vi "dI-dV(V)_MFLI_MF-MD_K3636B_measureX_PK_V4.0_withaveraging_copy.vi"() -> ()   [LabVIEW 2016]
uses:
  Labview Drivers/MFLI/LabOneLabVIEW-22.02.26577/LabOneLabVIEW-22.02.26577/Zurich Instruments LabOne/Public/Data/ziTypeDemodSampleSingle.ctl
  Application/Labview Drivers/Keithley 2600 Series/Public/Configure/Source/Configure Source (Limit).vi
  Application/Labview Drivers/Keithley 2600 Series/Public/Configure/Source/Configure Source (Range).vi
  Labview Drivers/MFLI/LabOneLabVIEW-22.02.26577/LabOneLabVIEW-22.02.26577/Zurich Instruments LabOne/Public/Configure/ziSetValueDouble.vi
  Labview Drivers/MFLI/LabOneLabVIEW-22.02.26577/LabOneLabVIEW-22.02.26577/Zurich Instruments LabOne/Public/Configure/ziGetValueDemodSampleEx.vi
  Labview Drivers/MFLI/LabOneLabVIEW-22.02.26577/LabOneLabVIEW-22.02.26577/Zurich Instruments LabOne/Zurich Instruments LabOne.lvlib
  Application/Labview Drivers/Keithley 2600 Series/Keithley 2600 Series.lvlib
panel:
  in  "MFLI Average":i32=50
  in  "MFLI Autorange":bool
  in  "Resistance used for DC (ohm)":dbl=2000000.0 format="%#_13g"
  in  "DC Current Limit (A)":dbl=0.001 format="%#_13g"
  in  "Keithley 2636B (channelA)":refnum<visa-resource-name>="GPIB0::26::INSTR"
  in  "DC Voltage averaging":dbl=10.0 format="%#_13g"
  out "Demod Sample Out 2":T1={"Timestamps (ticks)"=44415505503230, "X (Vrms)"=5.270432882217543e-11, "Y (Vrms)"=-1.265296628024292e-11, "Osc Phase (deg)"=0.033939324931969814, "Freq (Hz)"=7.919000069023241, "DIO"=0, "AuxIn0 (V)"=-0.16198342631105334, "AuxIn1 (V)"=0.0003336581285111606, "Trigger"=768}
  out "Demod Sample Out":T1={"Timestamps (ticks)"=44415354724350, "X (Vrms)"=9.977186384940147e-06, "Y (Vrms)"=-1.8750293191901917e-06, "Osc Phase (deg)"=0.8527015704659308, "Freq (Hz)"=7.919000069023241, "DIO"=0, "AuxIn0 (V)"=-0.15897133780526929, "AuxIn1 (V)"=0.0006673162570223212, "Trigger"=768}
  out "Vset (V)":dbl=-0.1590000000000001
  in  "stop":bool
  out "Time(s)":dbl=10295.486
  in  "Delay (s)":dbl=6.0
  out "dI/dV (S)":dbl=5.2300295748635186e-06
  out "dV (V)":dbl=1.0020577839232101e-05
  out "dI (A)":dbl=5.240791845640586e-11
  in  "MFLI Address":string="DEV4382"
  out "DC Voltage (V)":dbl=-0.001546351334
  in  "Folder":path=path "D:/Pranava/Data/STS/MA1981"
  out "dI/dV vs DC Bias (V)":cluster{dbl, "Field Reading":dbl}[](graph)=[{0.0015585960000000002, "Field Reading"=5.212882447768198e-06}, {0.0015574051580000002, "Field Reading"=5.216230609910891e-06}, {0.0015450042150000002, "Field Reading"=5.332655316612814e-06}, {0.0015402479659999998, "Field Reading"=5.179942635058783e-06}, {0.0015287444169999997, "Field Reading"=5.153653359756601e-06}, {0.001514132563, "Field Reading"=5.234083799441694e-06}, {0.0015012987609999999, "Field Reading"=5.216915331215124e-06}, {0.0014921046859999998, "Field Reading"=5.128533572067999e-06}, {0.0014823273930000002, "Field Reading"=5.2816317007055765e-06}, {0.001478375837, "Field Reading"=5.309228436563942e-06}, {0.0014697416179999998, "Field Reading"=5.180384733305549e-06}, {0.0014605146869999999, "Field Reading"=5.2437829272833834e-06}, {0.0014511105549999998, "Field Reading"=5.323573484146637e-06}, {0.001437617793, "Field Reading"=5.109135170585618e-06}, {0.001431351602, "Field Reading"=5.222537194595299e-06}, {0.001421562924, "Field Reading"=5.351572743051557e-06}, {0.001413336557, "Field Reading"=5.063485699973886e-06}, {0.0014017247129999998, "Field Reading"=5.245483958292874e-06}, {0.0013937929030000001, "Field Reading"=5.1726434044429675e-06}, {0.0013873947600000001, "Field Reading"=5.096425884973556e-06}, {0.001380029772, "Field Reading"=5.129762465549782e-06}, {0.001368911084, "Field Reading"=5.239923555898619e-06}, {0.0013538410640000001, "Field Reading"=5.163937857982776e-06}, {0.0013435478299999998, "Field Reading"=5.162252456443757e-06}, {0.001337313305, "Field Reading"=5.223196703884617e-06}, {0.001328354277, "Field Reading"=5.222236292899867e-06}, {0.0013159523039999999, "Field Reading"=5.1470185548003235e-06}, {0.001310923057, "Field Reading"=5.145583384677281e-06}, {0.0012968772209999999, "Field Reading"=5.240599601304534e-06}, {0.001288045918, "Field Reading"=5.163933072768467e-06}, {0.0012790827819999999, "Field Reading"=5.218772714395967e-06}, {0.001270189151, "Field Reading"=5.131294212056359e-06}, {0.0012604713519999999, "Field Reading"=5.257367658025543e-06}, {0.0012476149280000002, "Field Reading"=5.220909699961693e-06}, {0.001237396012, "Field Reading"=5.140651302506761e-06}, {0.001230543541, "Field Reading"=5.124508459293327e-06}, {0.001218331822, "Field Reading"=5.362041844273692e-06}, {0.0012103427570000001, "Field Reading"=5.20364900229283e-06}, {0.00119896285, "Field Reading"=5.1670228340471055e-06}, {0.001187731118, "Field Reading"=5.199330321545562e-06}, {0.001176843414, "Field Reading"=5.163000252164968e-06}, {0.0011673957599999999, "Field Reading"=5.258701429432347e-06}, {0.001154014224, "Field Reading"=5.10955819872187e-06}, {0.001144962631, "Field Reading"=5.186033499821924e-06}, {0.0011360305839999997, "Field Reading"=5.204922243103885e-06}, {0.001123625668, "Field Reading"=5.206409404883258e-06}, {0.001120136697, "Field Reading"=5.100767560564291e-06}, {0.0011074265280000002, "Field Reading"=5.284248912836877e-06}, {0.001101597482, "Field Reading"=5.244102839871407e-06}, {0.0010930735149999999, "Field Reading"=5.060130647735595e-06}, {0.00108164638, "Field Reading"=5.255631269341345e-06}, {0.0010743437349999998, "Field Reading"=5.175892983896831e-06}, {0.0010675353839999999, "Field Reading"=5.0722612270562495e-06}, {0.001054919456, "Field Reading"=5.094669979887855e-06}, {0.0010452565929999998, "Field Reading"=5.267795249536569e-06}, {0.001031836103, "Field Reading"=5.265208682667313e-06}, {0.0010242623, "Field Reading"=5.045017477422646e-06}, {0.0010142625369999997, "Field Reading"=5.226795793118276e-06}, {0.0010031751420000001, "Field Reading"=5.185351845821973e-06}, {0.0009973647708, "Field Reading"=5.060624976005092e-06}, {0.0009838739573000002, "Field Reading"=5.2115616231347515e-06}, {0.0009721488018999998, "Field Reading"=5.197797933274164e-06}, {0.0009623698433000001, "Field Reading"=5.117412900401103e-06}, {0.0009549787590000001, "Field Reading"=5.271050163095251e-06}, {0.0009425562177000002, "Field Reading"=5.089099697431323e-06}, {0.0009346050482, "Field Reading"=5.111858075720655e-06}, {0.0009278794926999999, "Field Reading"=5.3141760004903695e-06}, {0.0009175378259, "Field Reading"=5.212813032258665e-06}, {0.0009050930221999999, "Field Reading"=5.059365897630443e-06}, {0.0008940022000999999, "Field Reading"=5.213020179523542e-06}, {0.0008868497982, "Field Reading"=5.132768541234761e-06}, {0.000873987177, "Field Reading"=5.098692604191086e-06}, {0.0008647336786000001, "Field Reading"=5.175803992441765e-06}, {0.0008578628752, "Field Reading"=5.1406902882042985e-06}, {0.0008497464350000001, "Field Reading"=5.05078774437629e-06}, {0.0008390847227, "Field Reading"=5.1318585897566e-06}, {0.0008281325092999999, "Field Reading"=5.2170721058417935e-06}, {0.0008151434625, "Field Reading"=5.107566285449003e-06}, {0.0008076430619000001, "Field Reading"=5.164789493877711e-06}, {0.0007973502912, "Field Reading"=5.158601322505396e-06}, {0.0007877470746000001, "Field Reading"=5.189469152531585e-06}, {0.0007773389743, "Field Reading"=5.14181572846548e-06}, {0.0007669253149, "Field Reading"=5.170477401651019e-06}, {0.000760976265, "Field Reading"=5.181551189549383e-06}, {0.0007507472970999998, "Field Reading"=5.057433412487052e-06}, {0.0007410885564999999, "Field Reading"=5.162974839927331e-06}, {0.0007292004295000001, "Field Reading"=5.011556140975368e-06}, {0.0007194136834, "Field Reading"=4.9838450640076085e-06}, {0.0007135791361, "Field Reading"=5.154973547848261e-06}, {0.0006967615573, "Field Reading"=5.03038308908581e-06}, {0.000689380425, "Field Reading"=5.093366243021106e-06}, {0.0006797753657, "Field Reading"=5.220980427689892e-06}, {0.0006690933893000001, "Field Reading"=5.170097458275576e-06}, {0.0006593942345, "Field Reading"=5.034565078574319e-06}, {0.0006506193482, "Field Reading"=5.105681476546405e-06}, {0.0006416821833, "Field Reading"=5.024705219958056e-06}, {0.0006323520569, "Field Reading"=4.953532342283896e-06}, {0.0006210674437, "Field Reading"=5.146446194103851e-06}, {0.000612110108, "Field Reading"=5.002860539008119e-06}, {0.0006066923645000001, "Field Reading"=5.074217976077293e-06}, {0.0005957508622999999, "Field Reading"=5.131789689717381e-06}, {0.0005878011297, "Field Reading"=5.029683330946868e-06}, {0.0005761504233, "Field Reading"=5.11172725110063e-06}, {0.0005670423507, "Field Reading"=5.107118773588902e-06}, {0.0005569050149000001, "Field Reading"=5.1384132711483826e-06}, {0.0005458119266000001, "Field Reading"=5.08384297892591e-06}, {0.0005355046890000001, "Field Reading"=5.093620352610237e-06}, {0.0005276686571000001, "Field Reading"=5.048726313588527e-06}, {0.0005185426334999999, "Field Reading"=5.075498514679321e-06}, {0.0005067231144, "Field Reading"=5.138500407754088e-06}, {0.0004948162036999999, "Field Reading"=5.027073842849706e-06}, {0.00048122387290000003, "Field Reading"=4.9539252396109215e-06}, {0.00046572792420000004, "Field Reading"=5.151812218488621e-06}, {0.00045947953489999994, "Field Reading"=4.950582656963335e-06}, {0.000445468369, "Field Reading"=4.9629727593660924e-06}, {0.0004401750617, "Field Reading"=5.051519455232895e-06}, {0.00043223039239999994, "Field Reading"=5.019196156384289e-06}, {0.0004232032377, "Field Reading"=4.94697119310911e-06}, {0.00041321338979999995, "Field Reading"=5.092621993737827e-06}, {0.0004034016058, "Field Reading"=4.990782456637394e-06}, {0.00039670261360000004, "Field Reading"=4.931564034186295e-06}, {0.0003856912156, "Field Reading"=5.063913615233599e-06}, {0.00037828765239999995, "Field Reading"=4.959076493831628e-06}, {0.0003654108648, "Field Reading"=4.942001769456485e-06}, {0.0003564179983, "Field Reading"=4.943059683805646e-06}, {0.0003448496602, "Field Reading"=5.061021337291975e-06}, {0.0003342153665, "Field Reading"=4.962105311306236e-06}, {0.00031997468719999997, "Field Reading"=4.958115153731525e-06}, {0.0003174061527, "Field Reading"=5.052077149363862e-06}, {0.00030943723679999994, "Field Reading"=5.022482636318309e-06}, {0.0003007305683, "Field Reading"=4.9404548837080885e-06}, {0.00030190959010000006, "Field Reading"=5.12599052873285e-06}, {0.00029767182939999996, "Field Reading"=5.061427695219931e-06}, {0.0002938496221, "Field Reading"=4.961002797275753e-06}, {0.0002942324896, "Field Reading"=4.997667540747505e-06}, {0.0002911029924, "Field Reading"=4.998246143263189e-06}, {0.00029061966530000003, "Field Reading"=4.874936282198858e-06}, {0.0002878678893, "Field Reading"=4.945715269810476e-06}, {0.0002867975508, "Field Reading"=4.9133629527670024e-06}, {0.00028573036690000006, "Field Reading"=4.893144587666293e-06}, {0.00028452140900000003, "Field Reading"=4.875665751251186e-06}, {0.0002834161798, "Field Reading"=5.079360496712192e-06}, {0.00028160637040000006, "Field Reading"=5.007521533204678e-06}, {0.0002811224678, "Field Reading"=4.924805631344254e-06}, {0.00027980614529999996, "Field Reading"=5.106190399281268e-06}, {0.0002788066627, "Field Reading"=4.844823933637827e-06}, {0.00027513684300000004, "Field Reading"=4.877487386939147e-06}, {0.0002751094989, "Field Reading"=5.130568358975792e-06}, {0.0002770056507, "Field Reading"=4.910252317479383e-06}, {0.0002740377688, "Field Reading"=4.91828105634253e-06}, {0.0002744576125, "Field Reading"=5.063549456040986e-06}, {0.000273565677, "Field Reading"=4.957638010447136e-06}, {0.00027306061410000006, "Field Reading"=4.8478668905451095e-06}, {0.00027274906920000003, "Field Reading"=4.941723235231379e-06}, {0.0002722230268, "Field Reading"=5.004517849170231e-06}, {0.00026886406329999996, "Field Reading"=5.053834268866553e-06}, {0.0002702039868, "Field Reading"=4.8971448061664295e-06}, {0.0002673067398, "Field Reading"=4.998281648792141e-06}, {0.000265224059, "Field Reading"=4.981678709227842e-06}, {0.000263136064, "Field Reading"=4.9192134482136055e-06}, {0.0002618700027, "Field Reading"=4.9900924422343446e-06}, {0.0002607757632, "Field Reading"=4.9731182600615145e-06}, {0.0002614684793, "Field Reading"=4.9651706769720485e-06}, {0.0002543950071, "Field Reading"=4.85797296980987e-06}, {0.00025601706349999995, "Field Reading"=5.09299564803883e-06}, {0.0002586727928, "Field Reading"=4.965292651389097e-06}, {0.0002556323698, "Field Reading"=4.884183884312142e-06}, {0.00025431311229999996, "Field Reading"=4.997385182279032e-06}, {0.00025044809499999996, "Field Reading"=5.019211928478028e-06}, {0.0002507661319, "Field Reading"=4.937951427360642e-06}, {0.0002510081258, "Field Reading"=4.8994028091176744e-06}, {0.00025157834610000003, "Field Reading"=4.985730939592976e-06}, {0.0002483814422, "Field Reading"=5.008256978579852e-06}, {0.0002491548718, "Field Reading"=4.84628280880189e-06}, {0.00024779964939999996, "Field Reading"=4.934620427736037e-06}, {0.0002508299596, "Field Reading"=5.0072086632078186e-06}, {0.00025395816289999995, "Field Reading"=4.9084106682470995e-06}, {0.00025132225789999997, "Field Reading"=4.944878519822289e-06}, {0.0002478955164, "Field Reading"=4.983315732357e-06}, {0.0002401456697, "Field Reading"=4.925776772650806e-06}, {0.00024057087699999997, "Field Reading"=4.900148864051101e-06}, {0.00024259634460000002, "Field Reading"=5.016737965983632e-06}, {0.00024119371040000004, "Field Reading"=4.92877647066814e-06}, {0.00024203818749999996, "Field Reading"=4.986158386025063e-06}, {0.0002389471333, "Field Reading"=5.071244593644083e-06}, {0.00023578064720000002, "Field Reading"=4.872811081315698e-06}, {0.0002349980021, "Field Reading"=4.9557467644540525e-06}, {0.0002338782788, "Field Reading"=4.9589795883211275e-06}, {0.00023276223830000003, "Field Reading"=4.915911669622956e-06}, {0.0002339464169, "Field Reading"=5.0517572841427514e-06}, {0.0002291230541, "Field Reading"=4.9983348170821855e-06}, {0.00023532344000000001, "Field Reading"=4.89916696056797e-06}, {0.000231172722, "Field Reading"=5.0018521435752904e-06}, {0.00023344581690000005, "Field Reading"=4.960175469759237e-06}, {0.00023390273549999999, "Field Reading"=4.922324835774928e-06}, {0.0002318276875, "Field Reading"=4.956047547302315e-06}, {0.00023070873549999998, "Field Reading"=5.000144029334506e-06}, {0.0002341953257, "Field Reading"=4.897702174267421e-06}, {0.00023502290980000003, "Field Reading"=4.9459135714112385e-06}, {0.0002315661343, "Field Reading"=4.959370643289493e-06}, {0.00023167244950000003, "Field Reading"=4.866081512643599e-06}, {0.00022608803649999996, "Field Reading"=4.998095480411182e-06}, {0.00022276199789999997, "Field Reading"=4.934863328881881e-06}, {0.0002177185807, "Field Reading"=4.9030032636491686e-06}, {0.00021895938689999995, "Field Reading"=4.99712182835159e-06}, {0.0002247147147, "Field Reading"=4.906002768658836e-06}, {0.0002212600755, "Field Reading"=4.9301492904391556e-06}, {0.00022089307739999998, "Field Reading"=4.982685462603845e-06}, {0.00021838672859999996, "Field Reading"=4.947920765175706e-06}, {0.0002169405181, "Field Reading"=4.984935453257683e-06}, {0.0002162225189, "Field Reading"=4.945848913887106e-06}, {0.0002137178307, "Field Reading"=4.834901127628823e-06}, {0.00021024266350000003, "Field Reading"=4.974452086953461e-06}, {0.00020948194659999999, "Field Reading"=4.940733164924528e-06}, {0.00021212496679999998, "Field Reading"=4.862027123797206e-06}, {0.0002145472199, "Field Reading"=4.9250619089678495e-06}, {0.00021186424739999998, "Field Reading"=5.081791494952473e-06}, {0.0002082551044, "Field Reading"=5.002568977187787e-06}, {0.00020902753289999998, "Field Reading"=4.885660343152446e-06}, {0.00020895457679999998, "Field Reading"=5.004214272174826e-06}, {0.00020902166219999998, "Field Reading"=4.9486848805562295e-06}, {0.0002083086354, "Field Reading"=4.907764457119857e-06}, {0.0002089729284, "Field Reading"=4.944267459201694e-06}, {0.000208217539, "Field Reading"=4.947532131127844e-06}, {0.00020817831929999999, "Field Reading"=4.951576229867545e-06}, {0.00020636030430000002, "Field Reading"=4.881562384397422e-06}, {0.0002037711294, "Field Reading"=5.076182806642664e-06}, {0.0002028536027, "Field Reading"=4.924215219155632e-06}, {0.0002049729501, "Field Reading"=4.857242073880349e-06}, {0.00019844096639999999, "Field Reading"=5.009119721150331e-06}, {0.00019924701529999998, "Field Reading"=5.088696106117204e-06}, {0.0001970827401, "Field Reading"=4.894971110190867e-06}, {0.0001970069332, "Field Reading"=4.874686506057052e-06}, {0.00019379337100000003, "Field Reading"=4.980897333063725e-06}, {0.00019435483929999999, "Field Reading"=5.007269300359349e-06}, {0.00019279088310000003, "Field Reading"=4.815480379946107e-06}, {0.00019516183009999998, "Field Reading"=5.066727612202478e-06}, {0.000192734518, "Field Reading"=4.9152476590165165e-06}, {0.00019027476180000002, "Field Reading"=4.8009886821899316e-06}, {0.0001908981097, "Field Reading"=4.883605267619772e-06}, {0.00018873806940000002, "Field Reading"=4.936898983403465e-06}, {0.0001853231482, "Field Reading"=4.890880105071754e-06}, {0.00018678303389999998, "Field Reading"=4.9115078741068344e-06}, {0.000190538496, "Field Reading"=4.957464697145397e-06}, {0.0001864277055, "Field Reading"=4.875485695719259e-06}, {0.0001860759852, "Field Reading"=4.889475721613814e-06}, {0.00019038316929999996, "Field Reading"=5.033244303948086e-06}, {0.0001902611782, "Field Reading"=4.9200053971829594e-06}, {0.0001879660266, "Field Reading"=4.823570430346995e-06}, {0.0001882274343, "Field Reading"=4.946207749529361e-06}, {0.0001810150767, "Field Reading"=5.0220919438163134e-06}, {0.0001822141966, "Field Reading"=4.839874894655532e-06}, {0.00018242664840000002, "Field Reading"=4.954784219018356e-06}, {0.0001797682964, "Field Reading"=4.925042404639321e-06}, {0.0001751496226, "Field Reading"=4.763933141224698e-06}, {0.0001736480306, "Field Reading"=5.0108619239961055e-06}, {0.0001718218669, "Field Reading"=4.860798055121756e-06}, {0.0001720665588, "Field Reading"=4.946247979011112e-06}, {0.00017074520000000002, "Field Reading"=4.939502708778343e-06}, {0.0001704195284, "Field Reading"=4.821673629303167e-06}, {0.0001715239112, "Field Reading"=4.9528680392628405e-06}, {0.00016753897599999998, "Field Reading"=4.9687238888274316e-06}, {0.0001661135421, "Field Reading"=4.797328848759588e-06}, {0.00016795838119999999, "Field Reading"=4.921499364277482e-06}, {0.00016647253410000001, "Field Reading"=4.95007913881613e-06}, {0.0001656870889, "Field Reading"=4.921608896120205e-06}, {0.0001654102804, "Field Reading"=4.901326780398538e-06}, {0.0001671791623, "Field Reading"=4.9392337983568085e-06}, {0.00016933976729999997, "Field Reading"=4.888455323704264e-06}, {0.0001617152635, "Field Reading"=4.869555853735234e-06}, {0.00015836269169999998, "Field Reading"=4.8995651782087675e-06}, {0.00016111930839999997, "Field Reading"=4.877014378881573e-06}, {0.0001572530582, "Field Reading"=4.864909996119802e-06}, {0.0001571868267, "Field Reading"=4.852346029119758e-06}, {0.00015334076700000002, "Field Reading"=5.039512574170353e-06}, {0.00015378453319999998, "Field Reading"=4.823134986446204e-06}, {0.0001534619543, "Field Reading"=4.819080264358249e-06}, {0.0001530743685, "Field Reading"=4.833249943062479e-06}, {0.0001526707122, "Field Reading"=4.9339228568998685e-06}, {0.00014990580209999998, "Field Reading"=4.746957053701507e-06}, {0.0001497378872, "Field Reading"=4.9153848384667285e-06}, {0.0001523377413, "Field Reading"=4.8944840329773795e-06}, {0.0001532884788, "Field Reading"=4.791427527897305e-06}, {0.0001505089318, "Field Reading"=4.868147039211884e-06}, {0.00015211351519999998, "Field Reading"=4.93533941505003e-06}, {0.0001507775457, "Field Reading"=4.852056277617582e-06}, {0.00014960643549999998, "Field Reading"=4.845794677550966e-06}, {0.0001516503838, "Field Reading"=5.015001951289549e-06}, {0.00014626213580000002, "Field Reading"=4.897707061981369e-06}, {0.0001456224249, "Field Reading"=4.906570166693808e-06}, {0.0001422588355, "Field Reading"=5.038674343078877e-06}, {0.00014249603469999997, "Field Reading"=4.841438898058855e-06}, {0.0001393736279, "Field Reading"=4.993006561322359e-06}, {0.0001384631506, "Field Reading"=4.942654053470765e-06}, {0.000140033048, "Field Reading"=4.946615607823212e-06}, {0.00013948677309999998, "Field Reading"=4.894923432437869e-06}, {0.0001385685263, "Field Reading"=4.958176292134781e-06}, {0.00013600199409999998, "Field Reading"=4.87165387183211e-06}, {0.0001381889418, "Field Reading"=4.9962152322398856e-06}, {0.0001342478441, "Field Reading"=4.962754210442425e-06}, {0.000130067769, "Field Reading"=4.804160259498173e-06}, {0.0001282095308, "Field Reading"=4.8989253604379875e-06}, {0.0001277063875, "Field Reading"=4.873228191469052e-06}, {0.00012654669809999999, "Field Reading"=4.817010624558279e-06}, {0.0001285189523, "Field Reading"=4.9337706507542525e-06}, {0.00012801710960000002, "Field Reading"=4.900506466739129e-06}, {0.00012757297689999997, "Field Reading"=4.816139254473648e-06}, {0.00012540435990000001, "Field Reading"=4.887678760671365e-06}, {0.0001241530151, "Field Reading"=4.9755783397738575e-06}, {0.00012158196960000002, "Field Reading"=4.751747167035884e-06}, {0.00012101287159999999, "Field Reading"=4.7975401421368665e-06}, {0.0001266064259, "Field Reading"=4.909957867016385e-06}, {0.0001176607497, "Field Reading"=4.883511098087177e-06}, {0.0001188277375, "Field Reading"=4.798634563883484e-06}, {0.0001195220765, "Field Reading"=4.883484289774239e-06}, {0.00011586728059999999, "Field Reading"=4.939867678037612e-06}, {0.0001141826813, "Field Reading"=4.811689578073808e-06}, {0.0001113538309, "Field Reading"=4.905159973706454e-06}, {0.00011083969959999999, "Field Reading"=4.920811369767922e-06}, {0.00011093647020000001, "Field Reading"=4.883895954504346e-06}, {0.0001120388694, "Field Reading"=4.8100365128914615e-06}, {0.0001078931275, "Field Reading"=4.904216136981448e-06}, {0.0001081162461, "Field Reading"=4.749687773037711e-06}, {0.00010949451, "Field Reading"=4.897173255414535e-06}, {0.00010645382939999999, "Field Reading"=4.872892501688329e-06}, {0.0001067106169, "Field Reading"=4.839287896965791e-06}, {0.00010543290970000001, "Field Reading"=4.8711942651728116e-06}, {0.00010182904720000002, "Field Reading"=4.930007454012828e-06}, {0.00010080054832999999, "Field Reading"=4.842925937130695e-06}, {9.986760449999998e-05, "Field Reading"=4.895520994481557e-06}, {9.95561829e-05, "Field Reading"=4.90240526635031e-06}, {9.749268155000001e-05, "Field Reading"=4.866444517772542e-06}, {9.670539371e-05, "Field Reading"=4.816024341102907e-06}, {9.484665844999999e-05, "Field Reading"=4.9083887842991435e-06}, {9.730285954e-05, "Field Reading"=4.849023398620808e-06}, {9.53019176e-05, "Field Reading"=4.782317681615887e-06}, {9.526366237000001e-05, "Field Reading"=4.883946534865466e-06}, {9.246455748999999e-05, "Field Reading"=4.806139048391928e-06}, {9.160858109e-05, "Field Reading"=4.782396224768919e-06}, {9.075377437000001e-05, "Field Reading"=4.872845783296105e-06}, {8.880116396e-05, "Field Reading"=4.857104395420089e-06}, {9.115566097e-05, "Field Reading"=4.728371035111875e-06}, {9.070757174e-05, "Field Reading"=4.835572832591118e-06}, {9.183714116999997e-05, "Field Reading"=4.84097871338037e-06}, {9.09538221e-05, "Field Reading"=4.802205777168018e-06}, {9.073960152999999e-05, "Field Reading"=4.8356088998293165e-06}, {9.184954323999999e-05, "Field Reading"=4.938660551949447e-06}, {8.732495716e-05, "Field Reading"=4.84917728174439e-06}, {8.871321208999998e-05, "Field Reading"=4.788302373415324e-06}, {8.949765098e-05, "Field Reading"=4.920705826208192e-06}, {8.944440370999999e-05, "Field Reading"=4.842580269503273e-06}, {8.843273518e-05, "Field Reading"=4.769096931373989e-06}, {8.632217477e-05, "Field Reading"=4.848830891249846e-06}, {8.106427848000001e-05, "Field Reading"=4.870525329812652e-06}, {7.956673404e-05, "Field Reading"=4.735894837194288e-06}, {7.755950312999999e-05, "Field Reading"=4.917887164548008e-06}, {7.879757123e-05, "Field Reading"=4.899784768950785e-06}, {8.234973146e-05, "Field Reading"=4.745306151203819e-06}, {8.130352096e-05, "Field Reading"=4.864012035821515e-06}, {7.902302850999999e-05, "Field Reading"=4.860927412670961e-06}, {7.839681235999999e-05, "Field Reading"=4.8257433740314396e-06}, {7.914806762e-05, "Field Reading"=4.941593172346331e-06}, {7.35923637e-05, "Field Reading"=4.857793972169302e-06}, {7.506179553e-05, "Field Reading"=4.753818859610119e-06}, {7.271061373e-05, "Field Reading"=4.7572535345756465e-06}, {7.393803989e-05, "Field Reading"=4.92575534758845e-06}, {6.746911402e-05, "Field Reading"=4.724134588064619e-06}, {6.955808251999999e-05, "Field Reading"=4.748768602620094e-06}, {7.052522193e-05, "Field Reading"=4.857841340864884e-06}, {6.951223723000002e-05, "Field Reading"=4.755390514338632e-06}, {6.539709277999999e-05, "Field Reading"=4.779388882048e-06}, {6.560886100999999e-05, "Field Reading"=4.891252911410044e-06}, {6.620706013e-05, "Field Reading"=4.721261199216204e-06}, {7.014292830000001e-05, "Field Reading"=4.696951032379622e-06}, {6.566702549e-05, "Field Reading"=4.786021162075938e-06}, {6.262627123e-05, "Field Reading"=4.7846236269608605e-06}, {6.198595476999998e-05, "Field Reading"=4.708808767569022e-06}, {5.846888745e-05, "Field Reading"=4.877434372294174e-06}, {5.825552057e-05, "Field Reading"=4.741400730714019e-06}, {5.620048377e-05, "Field Reading"=4.7797911168917604e-06}, {5.532170881e-05, "Field Reading"=4.839903069614195e-06}, {5.457549811e-05, "Field Reading"=4.797886754081175e-06}, {5.383098525e-05, "Field Reading"=4.770331636485864e-06}, {5.301653957999999e-05, "Field Reading"=4.877322868099732e-06}, {5.118765065e-05, "Field Reading"=4.717065948116073e-06}, {4.8170082310000004e-05, "Field Reading"=4.822259445843764e-06}, {4.5293744170000004e-05, "Field Reading"=4.815021279603292e-06}, {4.5668965380000004e-05, "Field Reading"=4.721998694615662e-06}, {4.437664489e-05, "Field Reading"=4.792010174769188e-06}, {4.301429581e-05, "Field Reading"=4.734759014289611e-06}, {4.208970993e-05, "Field Reading"=4.735850505895278e-06}, {3.755228548e-05, "Field Reading"=4.736981699309213e-06}, {3.8500232229999995e-05, "Field Reading"=4.851553781062291e-06}, {3.819060886000001e-05, "Field Reading"=4.715246506487222e-06}, {3.622047326e-05, "Field Reading"=4.663722865227953e-06}, {3.860824052e-05, "Field Reading"=4.764220009110558e-06}, {3.6044396590000006e-05, "Field Reading"=4.6477482878450466e-06}, {3.5565082460000006e-05, "Field Reading"=4.669862811648826e-06}, {3.381357103e-05, "Field Reading"=4.818180802714367e-06}, {3.179851405e-05, "Field Reading"=4.7361650243783e-06}, {2.9543724580000005e-05, "Field Reading"=4.677349074539626e-06}, {3.0224895210000005e-05, "Field Reading"=4.714379581298665e-06}, {2.918087164e-05, "Field Reading"=4.700573274680611e-06}, {2.8331305870000003e-05, "Field Reading"=4.571010856347274e-06}, {3.1173776610000003e-05, "Field Reading"=4.765291030022407e-06}, {2.805833296e-05, "Field Reading"=4.634818744529924e-06}, {2.866522715e-05, "Field Reading"=4.664830027891397e-06}, {2.8043029080000004e-05, "Field Reading"=4.792073076465266e-06}, {2.8040046609999994e-05, "Field Reading"=4.561123598693244e-06}, {2.510323216e-05, "Field Reading"=4.676153087996679e-06}, {2.277465652e-05, "Field Reading"=4.750628279934504e-06}, {2.2132117029999997e-05, "Field Reading"=4.633857198555041e-06}, {2.1437448759999997e-05, "Field Reading"=4.808745410882639e-06}, {2.1435030829999998e-05, "Field Reading"=4.7432762017858555e-06}, {2.22151342e-05, "Field Reading"=4.547205478043862e-06}, {2.3747934820000002e-05, "Field Reading"=4.624482983847606e-06}, {2.0498608499999997e-05, "Field Reading"=4.77341802105419e-06}, {2.3111715039999998e-05, "Field Reading"=4.758430065244465e-06}, {1.7393441650000003e-05, "Field Reading"=4.61634531452973e-06}, {1.755487899e-05, "Field Reading"=4.746401122140536e-06}, {1.6348042389999998e-05, "Field Reading"=4.704526532506162e-06}, {1.1925376789999998e-05, "Field Reading"=4.629846448153783e-06}, {1.7048293849999997e-05, "Field Reading"=4.592624094847494e-06}, {2.0278471089999998e-05, "Field Reading"=4.7523372603449324e-06}, {1.530066937e-05, "Field Reading"=4.601270940973365e-06}, {1.367525143e-05, "Field Reading"=4.6068515331715175e-06}, {1.099021055e-05, "Field Reading"=4.75650742193199e-06}, {1.317791647e-05, "Field Reading"=4.701040381727732e-06}, {1.137035864e-05, "Field Reading"=4.564750535130856e-06}, {6.488639689e-06, "Field Reading"=4.642003796593938e-06}, {8.425750784e-06, "Field Reading"=4.760027752891156e-06}, {7.306599373e-06, "Field Reading"=4.677374890984702e-06}, {8.701853705999998e-06, "Field Reading"=4.6912809984400965e-06}, {6.435453782e-06, "Field Reading"=4.72849428483782e-06}, {7.050634869e-06, "Field Reading"=4.545286841401398e-06}, {5.409731695999999e-06, "Field Reading"=4.682616890803659e-06}, {3.6890269889999997e-06, "Field Reading"=4.685677534152445e-06}, {5.0219369668e-07, "Field Reading"=4.562090792568658e-06}, {-3.40297825e-06, "Field Reading"=4.632645251962042e-06}, {-5.289957015000001e-06, "Field Reading"=4.684879183507982e-06}, {-1.0393159886999999e-05, "Field Reading"=4.7635460208981724e-06}, {-1.0867331407e-05, "Field Reading"=4.60567497197616e-06}, {-8.114632888999999e-06, "Field Reading"=4.71369734429011e-06}, {-1.0046642844999998e-05, "Field Reading"=4.802784280322882e-06}, {-1.0739785270000001e-05, "Field Reading"=4.674013425871309e-06}, {-9.918879027000002e-06, "Field Reading"=4.598277331960627e-06}, {-1.2680818210000001e-05, "Field Reading"=4.840803450182356e-06}, {-1.2337483649999997e-05, "Field Reading"=4.699075789244665e-06}, {-1.492499169e-05, "Field Reading"=4.6497733083637245e-06}, {-1.837025698e-05, "Field Reading"=4.729641809667418e-06}, {-1.837567613e-05, "Field Reading"=4.743426189990536e-06}, {-1.803976568e-05, "Field Reading"=4.766191820912417e-06}, {-1.661530107e-05, "Field Reading"=4.669063564441461e-06}, {-1.518338375e-05, "Field Reading"=4.790402973338145e-06}, {-1.874195388e-05, "Field Reading"=4.726946615918107e-06}, {-2.2110058750000002e-05, "Field Reading"=4.609760378639644e-06}, {-2.2223906890000004e-05, "Field Reading"=4.803727491043077e-06}, {-2.2361732149999995e-05, "Field Reading"=4.726618184206764e-06}, {-2.3243038079999997e-05, "Field Reading"=4.62776103133122e-06}, {-2.5348616029999996e-05, "Field Reading"=4.78687873151144e-06}, {-2.605009238e-05, "Field Reading"=4.7925781872195825e-06}, {-2.711371921e-05, "Field Reading"=4.691621219442809e-06}, {-3.0039624419999998e-05, "Field Reading"=4.768801454600894e-06}, {-3.032334365e-05, "Field Reading"=4.762254612680697e-06}, {-3.074537229e-05, "Field Reading"=4.666274811765254e-06}, {-3.205352141e-05, "Field Reading"=4.775540086844793e-06}, {-3.1819319639999996e-05, "Field Reading"=4.725256153010854e-06}, {-3.223117208e-05, "Field Reading"=4.685998240684017e-06}, {-3.306954764e-05, "Field Reading"=4.82419417331407e-06}, {-3.472388397e-05, "Field Reading"=4.700945395196224e-06}, {-3.390690613999999e-05, "Field Reading"=4.667208323265677e-06}, {-3.6127962869999995e-05, "Field Reading"=4.853612001333085e-06}, {-3.692851922e-05, "Field Reading"=4.820563596580844e-06}, {-3.4228449940000004e-05, "Field Reading"=4.6225526362834114e-06}, {-3.770542853000001e-05, "Field Reading"=4.846307983585725e-06}, {-3.79869552e-05, "Field Reading"=4.854396892831033e-06}, {-4.095033242e-05, "Field Reading"=4.699787617710059e-06}, {-4.823583271000001e-05, "Field Reading"=4.7700094914127175e-06}, {-4.9981673050000005e-05, "Field Reading"=4.901886861311712e-06}, {-5.0366489030000006e-05, "Field Reading"=4.78444184453287e-06}, {-5.577114127e-05, "Field Reading"=4.738973100130575e-06}, {-5.368836373e-05, "Field Reading"=4.834285431277693e-06}, {-5.0545001909999995e-05, "Field Reading"=4.819784434010677e-06}, {-5.4675879500000003e-05, "Field Reading"=4.749373545656933e-06}, {-5.238342667e-05, "Field Reading"=4.91125104520127e-06}, {-5.683902155e-05, "Field Reading"=4.880129778420983e-06}, {-5.9592172610000005e-05, "Field Reading"=4.682473140709441e-06}, {-5.695146908e-05, "Field Reading"=4.826823723942794e-06}, {-5.986472161e-05, "Field Reading"=4.881031226984114e-06}, {-5.933033811000001e-05, "Field Reading"=4.809809445323146e-06}, {-6.3270004e-05, "Field Reading"=4.783970652516035e-06}, {-6.37913185e-05, "Field Reading"=4.85208047461519e-06}, {-6.295688408e-05, "Field Reading"=4.831385705861522e-06}, {-6.37643121e-05, "Field Reading"=4.751279075872532e-06}, {-6.528071745999999e-05, "Field Reading"=4.789512599845752e-06}, {-6.572804258e-05, "Field Reading"=4.767678345285178e-06}, {-6.84112218e-05, "Field Reading"=4.748842317404716e-06}, {-6.986057466e-05, "Field Reading"=4.860375853500298e-06}, {-7.284461469999999e-05, "Field Reading"=4.857764041668459e-06}, {-7.201405843000002e-05, "Field Reading"=4.841616155301518e-06}, {-7.437271014e-05, "Field Reading"=4.951991735557716e-06}, {-7.377741069e-05, "Field Reading"=4.815681253298824e-06}, {-7.740000445e-05, "Field Reading"=4.764468793745882e-06}, {-7.677478724e-05, "Field Reading"=4.873097987530524e-06}, {-7.781783334e-05, "Field Reading"=4.879411037229003e-06}, {-7.928116099e-05, "Field Reading"=4.818221861187895e-06}, {-7.917427167000001e-05, "Field Reading"=4.7919995043713764e-06}, {-7.852179983e-05, "Field Reading"=4.848169128268572e-06}, {-8.013535898e-05, "Field Reading"=4.7928470263926635e-06}, {-8.295607142000001e-05, "Field Reading"=4.820993349321019e-06}, {-8.247293961e-05, "Field Reading"=4.862732069589896e-06}, {-8.256623848e-05, "Field Reading"=4.791331170200719e-06}, {-8.370277875999999e-05, "Field Reading"=4.76181607475673e-06}, {-8.313302626e-05, "Field Reading"=4.950509052648055e-06}, {-8.544345127e-05, "Field Reading"=4.822027270543052e-06}, {-8.734303456e-05, "Field Reading"=4.922228713524889e-06}, {-8.730288378e-05, "Field Reading"=4.89989433337585e-06}, {-8.591255538999997e-05, "Field Reading"=4.779526697645609e-06}, {-9.085826103e-05, "Field Reading"=4.828814113805192e-06}, {-9.332571967e-05, "Field Reading"=4.901956866410554e-06}, {-9.345128474999998e-05, "Field Reading"=4.743221964144835e-06}, {-9.69037451e-05, "Field Reading"=4.847755432884251e-06}, {-9.547603756e-05, "Field Reading"=4.913137786186926e-06}, {-9.600902607999998e-05, "Field Reading"=4.753209775625206e-06}, {-9.271150327999999e-05, "Field Reading"=4.845337981057381e-06}, {-9.343950212000002e-05, "Field Reading"=4.945730143222265e-06}, {-9.53463949e-05, "Field Reading"=4.80062443212388e-06}, {-0.0001015214734, "Field Reading"=4.828313984516348e-06}, {-0.00010001675014, "Field Reading"=4.840390994932813e-06}, {-0.00010415952279999999, "Field Reading"=4.883767730619671e-06}, {-0.00010371905029999998, "Field Reading"=4.784283127441888e-06}, {-0.0001028695944, "Field Reading"=4.861506167459943e-06}, {-0.0001033766188, "Field Reading"=4.879528858466649e-06}, {-0.0001063672262, "Field Reading"=4.8414560604898955e-06}, {-0.0001045547057, "Field Reading"=4.87190369506038e-06}, {-0.0001042664122, "Field Reading"=4.968715121647332e-06}, {-0.0001054147433, "Field Reading"=4.853494528088201e-06}, {-0.0001071952584, "Field Reading"=4.83710682936615e-06}, {-0.0001092127829, "Field Reading"=4.9984963839210964e-06}, {-0.00010955615890000002, "Field Reading"=4.835399256557216e-06}, {-0.0001136279278, "Field Reading"=4.8626796742048894e-06}, {-0.00011374520550000002, "Field Reading"=5.036428198418718e-06}, {-0.00011331882999999999, "Field Reading"=4.936012284236446e-06}, {-0.0001150368297, "Field Reading"=4.869184883771071e-06}, {-0.0001139767833, "Field Reading"=4.911133717157862e-06}, {-0.0001150277045, "Field Reading"=4.995378373509222e-06}, {-0.0001187680831, "Field Reading"=4.783534391276407e-06}, {-0.00011740960130000001, "Field Reading"=4.916573997702706e-06}, {-0.0001225845139, "Field Reading"=5.042910883756337e-06}, {-0.00011856547280000001, "Field Reading"=4.832450915743806e-06}, {-0.0001214604006, "Field Reading"=4.991365163532125e-06}, {-0.0001241289886, "Field Reading"=4.934960772695198e-06}, {-0.00012270521900000002, "Field Reading"=4.888916311299046e-06}, {-0.00012391270860000002, "Field Reading"=4.8587964547779515e-06}, {-0.0001195415477, "Field Reading"=4.9710248629871425e-06}, {-0.0001213979617, "Field Reading"=4.851304714372487e-06}, {-0.00012414684229999998, "Field Reading"=4.826383074703894e-06}, {-0.0001257041447, "Field Reading"=4.96104634502291e-06}, {-0.000125183388, "Field Reading"=4.832249955116556e-06}, {-0.0001264256123, "Field Reading"=4.827993270433017e-06}, {-0.0001281341687, "Field Reading"=4.845378145013522e-06}, {-0.0001316907196, "Field Reading"=4.814961510290109e-06}, {-0.00013301548720000002, "Field Reading"=4.868170216533334e-06}, {-0.0001347442147, "Field Reading"=4.876294486794686e-06}, {-0.00013342142569999999, "Field Reading"=4.8259227534413115e-06}, {-0.0001367939081, "Field Reading"=4.840813159944957e-06}, {-0.0001367364724, "Field Reading"=4.882918852609687e-06}, {-0.0001379637924, "Field Reading"=4.885810453079916e-06}, {-0.0001387770884, "Field Reading"=4.937936098650324e-06}, {-0.0001405413668, "Field Reading"=4.980024039648681e-06}, {-0.0001400988895, "Field Reading"=4.895459783924004e-06}, {-0.000142287619, "Field Reading"=4.8390950561635416e-06}, {-0.0001447666679, "Field Reading"=5.001285304427504e-06}, {-0.0001470502064, "Field Reading"=4.964619590011058e-06}, {-0.0001485476949, "Field Reading"=4.799336510476935e-06}, {-0.0001480069267, "Field Reading"=5.024152792673121e-06}, {-0.00014553432699999997, "Field Reading"=5.00063141485359e-06}, {-0.00014863931279999998, "Field Reading"=4.859645179729335e-06}, {-0.0001506756082, "Field Reading"=4.8584763607338684e-06}, {-0.00015127663869999997, "Field Reading"=4.966438997563061e-06}, {-0.0001502393465, "Field Reading"=4.882523728639168e-06}, {-0.00015608441020000002, "Field Reading"=4.8790807539698014e-06}, {-0.0001537408625, "Field Reading"=4.9869370403090715e-06}, {-0.00015621910479999998, "Field Reading"=4.9008670269971115e-06}, {-0.00015672279690000002, "Field Reading"=4.882772434314843e-06}, {-0.0001598139307, "Field Reading"=5.011060749850388e-06}, {-0.0001601735801, "Field Reading"=4.87416310643747e-06}, {-0.000164314445, "Field Reading"=4.844201723136302e-06}, {-0.00015973671600000002, "Field Reading"=4.968838976753908e-06}, {-0.00016110897410000002, "Field Reading"=4.94237926163908e-06}, {-0.0001620216554, "Field Reading"=4.856244073837624e-06}, {-0.00016276033009999998, "Field Reading"=4.991709572305193e-06}, {-0.0001639181067, "Field Reading"=4.928569916264607e-06}, {-0.0001630226579, "Field Reading"=4.848530003638687e-06}, {-0.0001650797194, "Field Reading"=4.8753767943300085e-06}, {-0.0001658435421, "Field Reading"=4.89080469308494e-06}, {-0.0001643149265, "Field Reading"=4.986686356065357e-06}, {-0.0001651210658, "Field Reading"=4.790948945068115e-06}, {-0.0001671750773, "Field Reading"=4.919877724419084e-06}, {-0.00016638534400000002, "Field Reading"=4.935501649545506e-06}, {-0.00017065239849999999, "Field Reading"=4.955421972007219e-06}, {-0.0001736781905, "Field Reading"=4.8531779378658535e-06}, {-0.0001736816985, "Field Reading"=5.003234559337716e-06}, {-0.0001737311257, "Field Reading"=5.0228027560307895e-06}, {-0.00017419027069999997, "Field Reading"=4.923199450317983e-06}, {-0.0001757971304, "Field Reading"=5.019512803480619e-06}, {-0.00017593388450000001, "Field Reading"=4.9252950650178685e-06}, {-0.0001785475909, "Field Reading"=4.914628630362796e-06}, {-0.00017475631799999998, "Field Reading"=4.947955486328483e-06}, {-0.000175440419, "Field Reading"=4.9902494486156124e-06}, {-0.0001782891858, "Field Reading"=4.867730798593561e-06}, {-0.00018028639760000003, "Field Reading"=4.922202677883459e-06}, {-0.00017992882279999997, "Field Reading"=4.933477246596789e-06}, {-0.00018170676730000002, "Field Reading"=4.993287460134706e-06}, {-0.0001797371788, "Field Reading"=4.8684938265728055e-06}, {-0.00018351286079999998, "Field Reading"=4.974973337174846e-06}, {-0.00018314473630000002, "Field Reading"=4.910785558476207e-06}, {-0.0001867373538, "Field Reading"=4.853281521687514e-06}, {-0.0001854661662, "Field Reading"=5.030350599029812e-06}, {-0.0001902296504, "Field Reading"=4.902878485803475e-06}, {-0.0001902163516, "Field Reading"=4.817175613225021e-06}, {-0.0001909858826, "Field Reading"=4.9231772973043074e-06}, {-0.0001888311253, "Field Reading"=4.961014627018192e-06}, {-0.000191011297, "Field Reading"=4.7253755103339444e-06}, {-0.00018934407970000003, "Field Reading"=4.970152317535769e-06}, {-0.00019268973489999997, "Field Reading"=4.998399922520928e-06}, {-0.0001971093161, "Field Reading"=4.799489193050714e-06}, {-0.0001948840729, "Field Reading"=4.9398100730201e-06}, {-0.0001974023024, "Field Reading"=4.928076816884317e-06}, {-0.00020158725319999998, "Field Reading"=4.858625188985831e-06}, {-0.00020056918130000002, "Field Reading"=4.83289160209355e-06}, {-0.00019842144009999998, "Field Reading"=4.927282286627908e-06}, {-0.000203712867, "Field Reading"=4.875834529699794e-06}, {-0.00020581847939999998, "Field Reading"=4.9635717127103e-06}, {-0.00020624803339999996, "Field Reading"=5.010995927419588e-06}, {-0.00020502449679999998, "Field Reading"=4.870397913609552e-06}, {-0.00020175262590000002, "Field Reading"=4.960007924177428e-06}, {-0.00020482674529999999, "Field Reading"=5.019287469026081e-06}, {-0.00020671416239999998, "Field Reading"=4.934628607672871e-06}, {-0.0002079022934, "Field Reading"=4.910356425740671e-06}, {-0.0002079855636, "Field Reading"=5.029435019210337e-06}, {-0.00021041971640000002, "Field Reading"=4.870643110486142e-06}, {-0.00021656574270000005, "Field Reading"=4.974232718446532e-06}, {-0.00021780882499999998, "Field Reading"=5.01772378918241e-06}, {-0.00021515812879999998, "Field Reading"=4.9589945697724385e-06}, {-0.00022031757799999998, "Field Reading"=4.9351364199465784e-06}, {-0.0002245504796, "Field Reading"=4.9655482265337455e-06}, {-0.0002230459688, "Field Reading"=4.882502095618291e-06}, {-0.00022401789770000002, "Field Reading"=5.083602544096488e-06}, {-0.00022467609390000001, "Field Reading"=4.951581091470307e-06}, {-0.00022363917970000003, "Field Reading"=4.903330694538623e-06}, {-0.00022324788319999996, "Field Reading"=5.027975997530168e-06}, {-0.00022229520200000002, "Field Reading"=4.965279867955158e-06}, {-0.0002244224962, "Field Reading"=4.93193195306129e-06}, {-0.00022490267000000006, "Field Reading"=4.9221599827113865e-06}, {-0.00022680169960000003, "Field Reading"=4.993097196593276e-06}, {-0.0002272118572, "Field Reading"=4.799721410652822e-06}, {-0.00022604578230000003, "Field Reading"=4.9961321560531256e-06}, {-0.00022901845559999997, "Field Reading"=4.8995887890516855e-06}, {-0.00023076743120000002, "Field Reading"=4.967625636060975e-06}, {-0.0002317895483, "Field Reading"=4.9345819595514824e-06}, {-0.0002281779504, "Field Reading"=5.020037320541726e-06}, {-0.0002255564484, "Field Reading"=4.905724607030067e-06}, {-0.00022763515520000003, "Field Reading"=4.93115140475374e-06}, {-0.0002271510647, "Field Reading"=5.007746221805023e-06}, {-0.00023191429219999996, "Field Reading"=4.936413146817249e-06}, {-0.00023031117060000003, "Field Reading"=4.95957980347047e-06}, {-0.00023519684359999993, "Field Reading"=5.097353174600031e-06}, {-0.00023872010520000002, "Field Reading"=4.925760726597818e-06}, {-0.0002385344042, "Field Reading"=5.060730426514436e-06}, {-0.00023817993579999997, "Field Reading"=4.950142718995509e-06}, {-0.0002400582004, "Field Reading"=4.989461667487861e-06}, {-0.00023962322800000002, "Field Reading"=4.988242389323803e-06}, {-0.00024244128890000004, "Field Reading"=4.9120960587507e-06}, {-0.00024435482499999997, "Field Reading"=5.071083358710323e-06}, {-0.0002445401272, "Field Reading"=4.9878699095593045e-06}, {-0.0002425280896, "Field Reading"=4.897510740372076e-06}, {-0.000245443773, "Field Reading"=4.9418042580938875e-06}, {-0.00024289763979999996, "Field Reading"=5.012759734846625e-06}, {-0.00024701041589999997, "Field Reading"=4.895512651738562e-06}, {-0.0002482376791, "Field Reading"=4.994235439436638e-06}, {-0.00025100000160000006, "Field Reading"=5.091849628818598e-06}, {-0.00025162067690000006, "Field Reading"=4.816178965276862e-06}, {-0.0002524568212, "Field Reading"=4.905063906558785e-06}, {-0.00025347157330000004, "Field Reading"=4.927295831023095e-06}, {-0.0002553450192, "Field Reading"=4.924381727493585e-06}, {-0.00025588715770000003, "Field Reading"=4.877405801996607e-06}, {-0.00025705109199999996, "Field Reading"=4.987744664863229e-06}, {-0.00025889091629999997, "Field Reading"=4.999516934634088e-06}, {-0.00026133597289999995, "Field Reading"=4.814074608228709e-06}, {-0.0002616743667, "Field Reading"=4.968088208333271e-06}, {-0.00026077061689999995, "Field Reading"=5.049206169421169e-06}, {-0.00025741090679999996, "Field Reading"=4.890088267334017e-06}, {-0.00025816587789999996, "Field Reading"=4.852141633290118e-06}, {-0.0002624854439, "Field Reading"=5.015462696499223e-06}, {-0.000262487167, "Field Reading"=4.9963401553680265e-06}, {-0.00026207301469999993, "Field Reading"=4.892155072396019e-06}, {-0.00026752334830000004, "Field Reading"=4.947321076648246e-06}, {-0.00026923098669999994, "Field Reading"=5.013503336141897e-06}, {-0.00026813510219999995, "Field Reading"=4.9579514406797565e-06}, {-0.0002707276849, "Field Reading"=5.006608248035885e-06}, {-0.000271572883, "Field Reading"=5.0360956569055115e-06}, {-0.0002710174498, "Field Reading"=4.897520666377915e-06}, {-0.0002731774588, "Field Reading"=5.064074316316541e-06}, {-0.0002780690979, "Field Reading"=5.0823397215452936e-06}, {-0.0002788758582, "Field Reading"=4.9378760543811635e-06}, {-0.0002784287958, "Field Reading"=4.960856755893159e-06}, {-0.00027599557969999993, "Field Reading"=4.985082217935568e-06}, {-0.0002765092654, "Field Reading"=4.92483569061321e-06}, {-0.00027859514600000004, "Field Reading"=4.961229608150725e-06}, {-0.00027678084349999995, "Field Reading"=5.060250046449556e-06}, {-0.0002825298153, "Field Reading"=4.9119589744350406e-06}, {-0.0002849377501, "Field Reading"=4.92275965309169e-06}, {-0.000284880009, "Field Reading"=4.949335806024827e-06}, {-0.00028733793380000003, "Field Reading"=5.0316626287091165e-06}, {-0.0002867615887, "Field Reading"=4.9335265059682825e-06}, {-0.0002924190922, "Field Reading"=4.890128181916824e-06}, {-0.0002945681472, "Field Reading"=5.008250654245932e-06}, {-0.0002976283469, "Field Reading"=4.961635038077422e-06}, {-0.00029519092290000005, "Field Reading"=4.960787809214015e-06}, {-0.00029613495299999997, "Field Reading"=4.988167340049741e-06}, {-0.00029512398679999995, "Field Reading"=4.9589184174218235e-06}, {-0.0002964883631, "Field Reading"=4.957530334649914e-06}, {-0.0003000837873, "Field Reading"=5.033307191177451e-06}, {-0.0002938337021, "Field Reading"=5.04065848442617e-06}, {-0.0002931883343, "Field Reading"=4.9050740613050535e-06}, {-0.00029422832350000007, "Field Reading"=5.060232482905171e-06}, {-0.00029664688260000005, "Field Reading"=5.030380727244262e-06}, {-0.00030187310150000006, "Field Reading"=4.952377051344779e-06}, {-0.0003043825608, "Field Reading"=5.023228471085851e-06}, {-0.0003057137295, "Field Reading"=4.900444685166495e-06}, {-0.00030089257499999996, "Field Reading"=4.946101786689578e-06}, {-0.0003113786794, "Field Reading"=5.084300910519531e-06}, {-0.00032223668969999996, "Field Reading"=4.994330858737399e-06}, {-0.00033392784100000003, "Field Reading"=4.953859919736779e-06}, {-0.0003471756814, "Field Reading"=5.012094227510514e-06}, {-0.00035279703319999995, "Field Reading"=5.023448568393265e-06}, {-0.00036158143350000004, "Field Reading"=5.017038370118495e-06}, {-0.0003741024157, "Field Reading"=4.917959028265907e-06}, {-0.000381320946, "Field Reading"=5.0914902236244285e-06}, {-0.0003916748116999999, "Field Reading"=4.934173614693229e-06}, {-0.0004021668189, "Field Reading"=5.023957695898678e-06}, {-0.0004145540834, "Field Reading"=5.10577905541954e-06}, {-0.00042390639810000006, "Field Reading"=4.972931537574091e-06}, {-0.00043903757680000005, "Field Reading"=5.066024659003688e-06}, {-0.00044719099830000004, "Field Reading"=4.956153047025073e-06}, {-0.0004590912252999999, "Field Reading"=4.916827999186417e-06}, {-0.00046671275400000006, "Field Reading"=5.0719076035403505e-06}, {-0.00047116624920000007, "Field Reading"=5.152616561831915e-06}, {-0.00048173658920000007, "Field Reading"=4.957428226582225e-06}, {-0.0004927236065, "Field Reading"=4.95890730463766e-06}, {-0.0005059940150000001, "Field Reading"=5.021245930108982e-06}, {-0.0005122142302, "Field Reading"=5.072757159544885e-06}, {-0.0005206584646000001, "Field Reading"=4.970204790038438e-06}, {-0.0005299131267, "Field Reading"=5.068094239911865e-06}, {-0.0005412704656, "Field Reading"=5.0601401206451095e-06}, {-0.0005477539899, "Field Reading"=4.9656250117263694e-06}, {-0.0005596067116, "Field Reading"=5.093245950316351e-06}, {-0.0005699488748, "Field Reading"=5.119750334199846e-06}, {-0.000576056378, "Field Reading"=4.957739280688305e-06}, {-0.0005843978603, "Field Reading"=5.161440130194121e-06}, {-0.000597673759, "Field Reading"=5.202231076171711e-06}, {-0.0006068362748000001, "Field Reading"=5.0392591769379724e-06}, {-0.0006189531396, "Field Reading"=5.1177996897173535e-06}, {-0.0006285573392, "Field Reading"=5.125956893468323e-06}, {-0.0006329261603, "Field Reading"=5.084175781597206e-06}, {-0.0006447240488, "Field Reading"=5.230396470046661e-06}, {-0.0006535849689999999, "Field Reading"=5.0810168435316025e-06}, {-0.0006645998212, "Field Reading"=5.078422469050681e-06}, {-0.0006750976782, "Field Reading"=5.040684708619909e-06}, {-0.0006855854399000001, "Field Reading"=5.03181559570935e-06}, {-0.0006967764944, "Field Reading"=4.954679495314898e-06}, {-0.0007049225316000001, "Field Reading"=5.154816477901861e-06}, {-0.0007162625897999999, "Field Reading"=5.158874570549062e-06}, {-0.0007239806694999999, "Field Reading"=5.071061901782406e-06}, {-0.0007331130817, "Field Reading"=5.010795685591322e-06}, {-0.0007419818590999999, "Field Reading"=5.2102811727313196e-06}, {-0.0007502761273, "Field Reading"=5.018813069176294e-06}, {-0.0007599115056999999, "Field Reading"=5.133425237761309e-06}, {-0.0007707157120000001, "Field Reading"=5.114208714413928e-06}, {-0.0007807984372, "Field Reading"=5.037646859503158e-06}, {-0.0007879471139, "Field Reading"=5.067297720714512e-06}, {-0.0007981297914999999, "Field Reading"=5.123245741655298e-06}, {-0.0008095023029999999, "Field Reading"=5.059430068249161e-06}, {-0.0008200094748, "Field Reading"=5.123493475865952e-06}, {-0.0008299359563, "Field Reading"=5.04566914012894e-06}, {-0.0008369431477999999, "Field Reading"=5.107175754398842e-06}, {-0.0008485186707, "Field Reading"=5.202859694236045e-06}, {-0.0008590784557000001, "Field Reading"=5.069454173919106e-06}, {-0.0008700617524, "Field Reading"=5.087833264071197e-06}, {-0.0008776299843999998, "Field Reading"=5.3128905441171286e-06}, {-0.0008900764041999999, "Field Reading"=5.103301068415403e-06}, {-0.0008999750202999998, "Field Reading"=5.0861681121922266e-06}, {-0.0009102758440000001, "Field Reading"=5.1661467417673335e-06}, {-0.0009196853784, "Field Reading"=5.216975040228609e-06}, {-0.0009272867204, "Field Reading"=5.140223380982685e-06}, {-0.0009358810563, "Field Reading"=5.2518119961604045e-06}, {-0.0009454736481999999, "Field Reading"=5.213379050805687e-06}, {-0.0009546322969, "Field Reading"=5.132058446056267e-06}, {-0.0009632817872, "Field Reading"=5.121294446126226e-06}, {-0.0009716990769, "Field Reading"=5.206005264365461e-06}, {-0.0009851204064000002, "Field Reading"=5.123111126234343e-06}, {-0.0009943402683, "Field Reading"=5.116359659781257e-06}, {-0.0010067216970000002, "Field Reading"=5.27627841380479e-06}, {-0.0010148327900000001, "Field Reading"=5.028827550078587e-06}, {-0.001025762721, "Field Reading"=5.144459810117704e-06}, {-0.0010326784560000001, "Field Reading"=5.191862128831841e-06}, {-0.001043699626, "Field Reading"=5.035948927928941e-06}, {-0.001054912697, "Field Reading"=4.958866058468105e-06}, {-0.001064482075, "Field Reading"=5.232511171078044e-06}, {-0.0010722596860000002, "Field Reading"=5.08887147339824e-06}, {-0.00107823511, "Field Reading"=5.186792603907487e-06}, {-0.0010857629759999999, "Field Reading"=5.199718605794547e-06}, {-0.0010958979920000001, "Field Reading"=5.0909550671886704e-06}, {-0.0011075895809999998, "Field Reading"=5.098393662664006e-06}, {-0.0011184980029999999, "Field Reading"=5.171784626132379e-06}, {-0.0011292710659999998, "Field Reading"=5.1198784502156515e-06}, {-0.0011375581109999999, "Field Reading"=5.146523729041635e-06}, {-0.0011478989030000001, "Field Reading"=5.174275635034944e-06}, {-0.001157514984, "Field Reading"=5.187903079054888e-06}, {-0.0011685873019999999, "Field Reading"=5.217256331800405e-06}, {-0.001178022049, "Field Reading"=5.243725243480134e-06}, {-0.001189132623, "Field Reading"=5.098473655248297e-06}, {-0.0012005239589999999, "Field Reading"=5.246472786347912e-06}, {-0.001206402097, "Field Reading"=5.106186589600339e-06}, {-0.001215912433, "Field Reading"=5.125419999241209e-06}, {-0.0012222433889999998, "Field Reading"=5.264091850209511e-06}, {-0.001231664633, "Field Reading"=5.22546287430241e-06}, {-0.001240368644, "Field Reading"=5.089727791251553e-06}, {-0.0012510612829999999, "Field Reading"=5.260545484383268e-06}, {-0.0012624410459999998, "Field Reading"=5.199345582618461e-06}, {-0.0012706160919999999, "Field Reading"=5.090910125684842e-06}, {-0.0012814257470000001, "Field Reading"=5.1816148757638386e-06}, {-0.001290177239, "Field Reading"=5.316826960967727e-06}, {-0.001297849333, "Field Reading"=5.145331634827164e-06}, {-0.001307548515, "Field Reading"=5.106261052461808e-06}, {-0.0013136461470000002, "Field Reading"=5.2241505571711345e-06}, {-0.0013298504859999998, "Field Reading"=5.094833960994427e-06}, {-0.0013343492960000002, "Field Reading"=5.195658311227608e-06}, {-0.0013423908540000002, "Field Reading"=5.208071102895085e-06}, {-0.0013545551500000002, "Field Reading"=5.112011471630385e-06}, {-0.001365369742, "Field Reading"=5.111532639075416e-06}, {-0.0013759780719999999, "Field Reading"=5.2968451957165945e-06}, {-0.0013868729889999999, "Field Reading"=5.10445336770952e-06}, {-0.0013952151590000002, "Field Reading"=5.058403178205962e-06}, {-0.0014040331420000004, "Field Reading"=5.199748882538133e-06}, {-0.001414297241, "Field Reading"=5.151600293499994e-06}, {-0.001420910145, "Field Reading"=5.130093365532128e-06}, {-0.001429313099, "Field Reading"=5.243315558683664e-06}, {-0.001442492003, "Field Reading"=5.142326549196296e-06}, {-0.0014528244219999997, "Field Reading"=5.103552630393455e-06}, {-0.001462907509, "Field Reading"=5.266178160896788e-06}, {-0.001471012299, "Field Reading"=5.178819219037773e-06}, {-0.001477868704, "Field Reading"=5.1626457603552485e-06}, {-0.0014887821000000002, "Field Reading"=5.241539581094897e-06}, {-0.0014994287450000002, "Field Reading"=5.327618898433515e-06}, {-0.0015072674289999999, "Field Reading"=5.271378421121128e-06}, {-0.0015181244219999999, "Field Reading"=5.0829399926303936e-06}, {-0.001526436894, "Field Reading"=5.167080826657878e-06}, {-0.0015375053659999998, "Field Reading"=5.30525412772834e-06}, {-0.001546351334, "Field Reading"=5.2300295748635186e-06}]
  out "data":dbl[](array[numeric])=[10295.486, -0.001546351334, 5.240791845640586e-11, 1.0020577839232101e-05, 5.2300295748635186e-06, -0.1590000000000001, -7.950000000000006e-08]
  in  "Nanovoltmeter 2182a VISA":refnum<visa-resource-name>="GPIB0::4::INSTR"
  in  "Step":dbl[](array[numeric])=[0.001, 0.001, 0.001] min=-3000.0 max=3000.0 format="%.1e"
  in  "To":dbl[](array[numeric])=[0.03, -0.03, -0.16] min=-3000.0 max=3000.0 format="%.1e"
  in  "From":dbl[](array[numeric])=[0.16, 0.03, -0.03] min=-3000.0 max=3000.0 format="%.1e"
  in  "file name":string="026_MA1981_Dev007_dI-dV_11uV_54pA_baseT_K2636sweep_7.919Hz_float_6T_90deg_50ave"
  out "File path":path=path "D:/Pranava/Data/STS/MA1981/026_MA1981_Dev007_dI-dV_11uV_54pA_baseT_K2636sweep_7.919Hz_float_6T_90deg_50ave.dat"
  # ".dat"
  # "Set Voltage (V)"
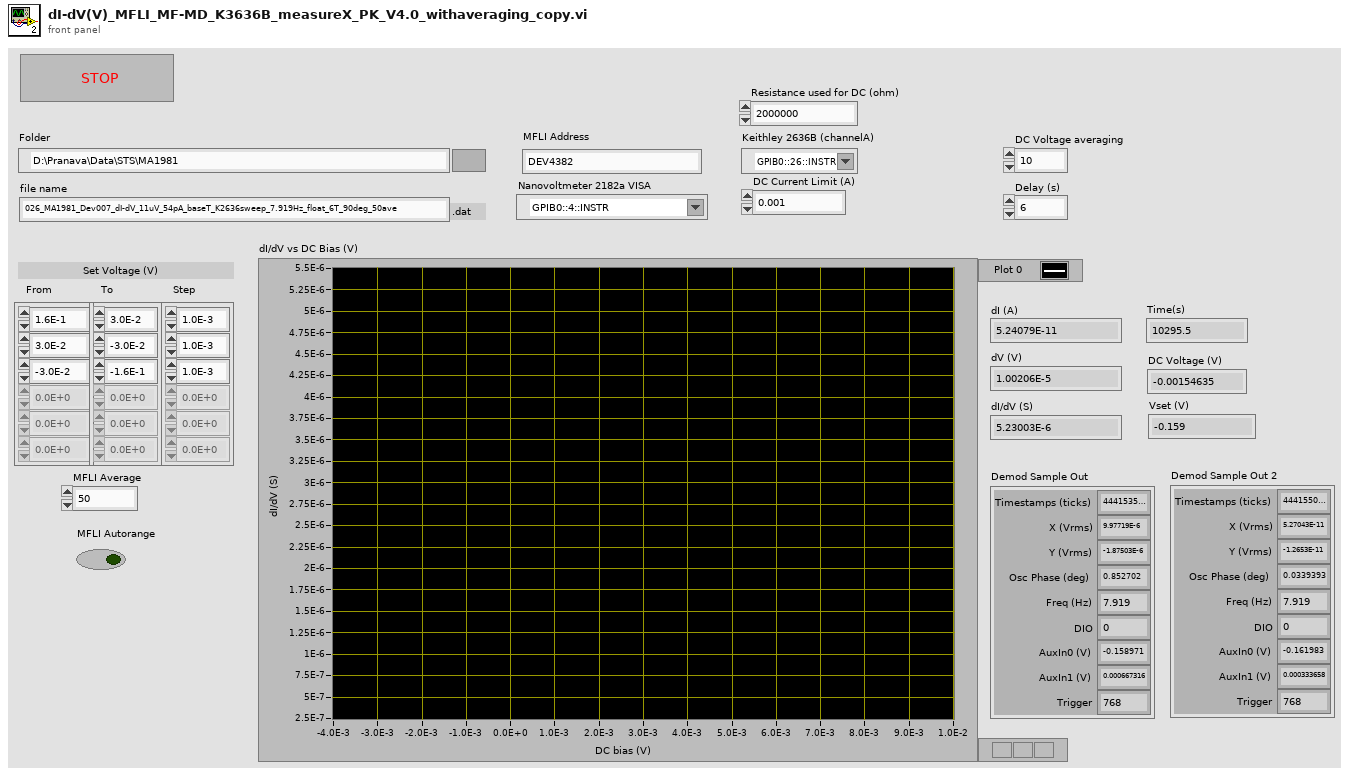
[diagram p1: front panel]
types:
  T1 = typedef "Zurich Instruments LabOne.lvlib/ziTypeDemodSampleSingle.ctl" = cluster{"Timestamps (ticks)":u64, "X (Vrms)":dbl, "Y (Vrms)":dbl, "Osc Phase (deg)":dbl, "Freq (Hz)":dbl, "DIO":u32, "AuxIn0 (V)":dbl, "AuxIn1 (V)":dbl, "Trigger":u32}
  T2 = enum16{"open", "replace", "create", "open or create", "replace or create", "replace or create with confirmation"}
  T3 = typedef "Zurich Instruments LabOne.lvlib/ziTypeHandle.ctl" = cluster{"handleValid":bool, "Conn":u64, "Path Prefix":string, "Handle":u64, "Connected":bool, "Clockbase(s)":dbl}
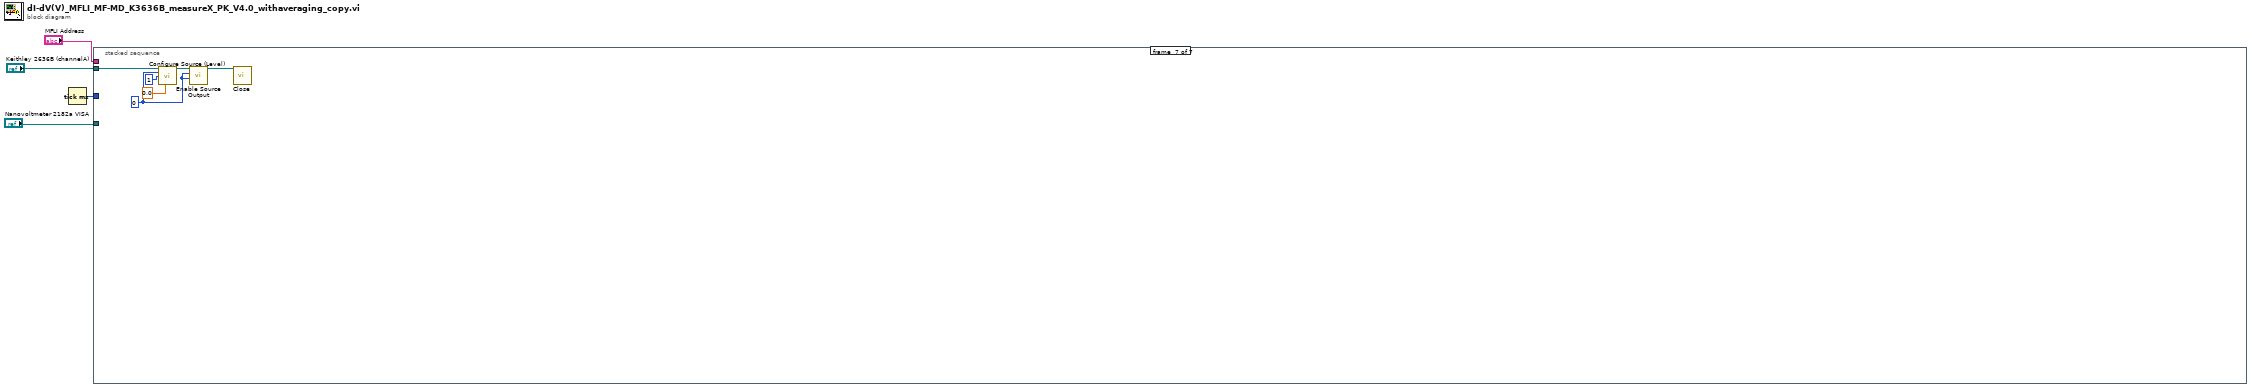
[diagram p0: block diagram]
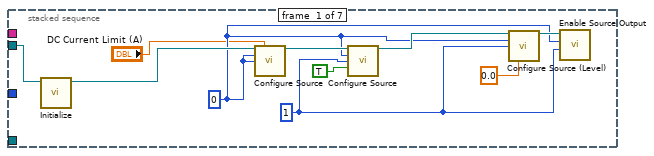
[diagram p2: hidden frame]
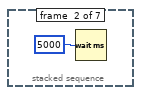
[diagram p3: hidden frame]
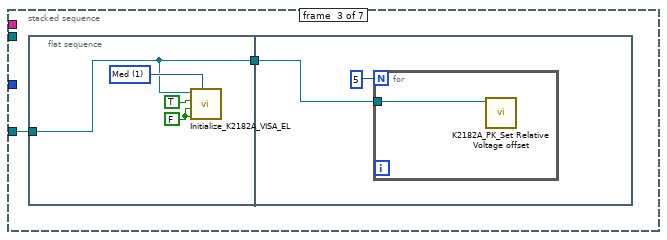
[diagram p4: hidden frame]
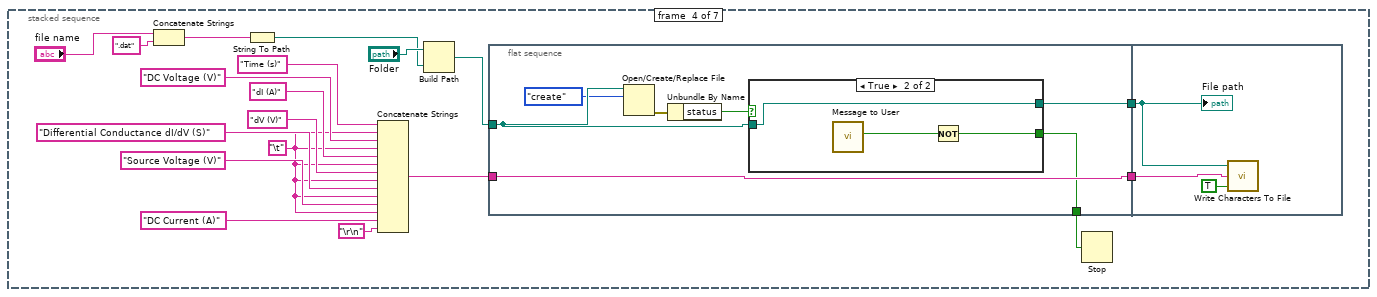
[diagram p5: hidden frame]
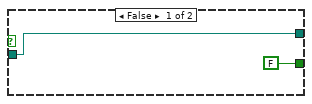
[diagram p6: hidden frame]
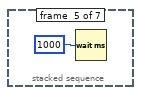
[diagram p7: hidden frame]
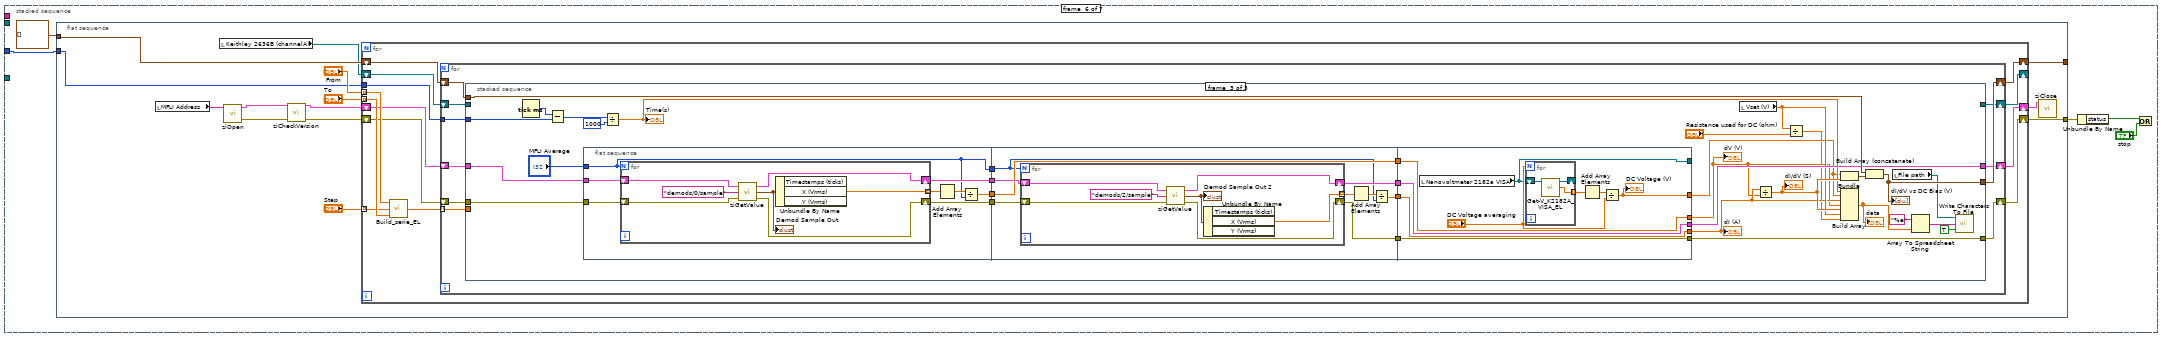
[diagram p8: hidden frame]
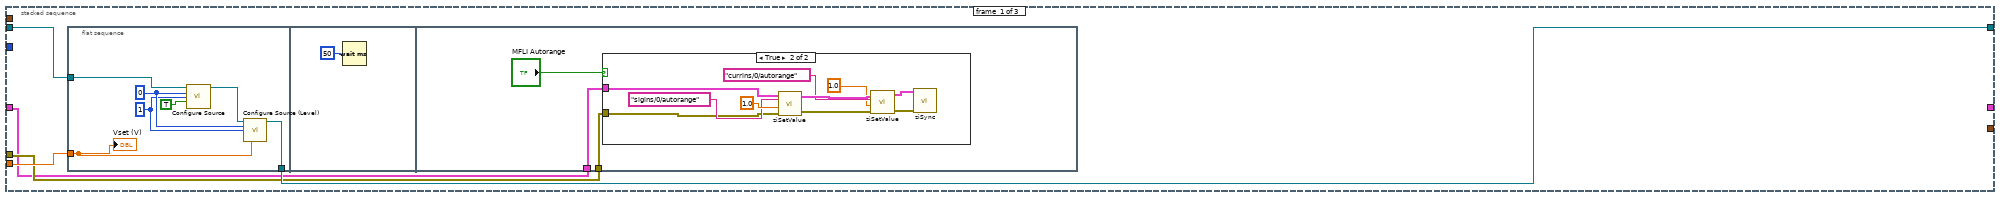
[diagram p9: hidden frame]
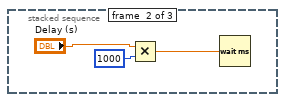
[diagram p11: hidden frame]
diagram:
  n1 = Tick Count (ms)() -> (millisecond timer value=w2:u32)
  n2 = stacked-sequence {
    tunnel: "Nanovoltmeter 2182a VISA" -> [_ _ w17 _ _ _ _]
    tunnel: "MFLI Address" -> [_ _ _ _ _ _ _]
    tunnel: w2 -> [_ _ _ _ _ w63 _]
    tunnel: "Keithley 2636B (channelA)" -> [w14 _ _ _ _ _ w209]
    frame #0 {
      w8 = 0
      w5 = 1
      n3 = call "Initialize.vi"("VISA resource name"=w14) -> ("VISA resource name out"=w13:refnum<visa-resource-name>)  [unwired: 9 in, 1 out]
      n4 = call-poly "Configure Source.vi"("VISA resource name"=w13, "Current Limit (0.1 A)"="DC Current Limit (A)", "Source Measure Unit Channel (0: Channel A)"=w8, "Limit Type (1: Voltage)"=w8) -> ("VISA resource name out"=w12:refnum<visa-resource-name>)  [unwired: 10 in, 1 out]
      n5 = call-poly "Configure Source.vi"("VISA resource name"=w12, "Source Measure Unit Channel (0: Channel A)"=w8, "Range Type (1: Voltage)"=w5, "Auto Range (T: Enable)"=TRUE) -> ("VISA resource name out"=w11:refnum<visa-resource-name>)  [unwired: 10 in, 1 out]
      n6 = call "Configure Source (Level).vi"("VISA resource name"=w11, "Source Measure Unit Channel (0: Channel A)"=w8, "Level Type (1: Voltage)"=w5, "Voltage Level (0 V)"=0.0) -> ("VISA resource name out"=w10:refnum<visa-resource-name>)  [unwired: 10 in, 1 out]
      n7 = call "Enable Source Output.vi"("Output Mode (0: Turn off)"=w5, "Source Measure Unit Channel (0: Channel A)"=w8, "VISA resource name"=w10) -> ()  [unwired: 7 in, 2 out]
    }
    frame #1 {
      n8 = Wait (ms)(milliseconds to wait=5000) -> ()  [unwired: 1 out]
    }
    frame #2 {
      n9 = flat-sequence {
        tunnel: w17 -> [w18]
        tunnel: [w18] -> w16
        tunnel: w16 -> [w22]
        frame #0 {
          w20 = u16 1 items=["Slow", "Med", "Fast"] ("Rate (NPLC)")
          w21 = FALSE ("Auto range?")
          n10 = call "Initialize_K2182A_VISA_EL.vi"("VISA address"=w18, "Auto range?"=TRUE, "Analog LPass\nFilter?"=w21, "DC\nFilter?"=w21, "Rate (NPLC)"=w20) -> ()  [unwired: 1 in, 1 out]
        }
        frame #1 {
          n11 = for {
            N: 5 ("Numeric") -> [_]
            tunnel: w22 -> [w24]
            n12 = call "K2182A_PK_Set Relative Voltage offset.vi"("VISA address"=w24) -> ()  [unwired: 11 in]
          }
        }
      }
    }
    frame #3 {
      w26 = "\t"
      n13 = Concatenate Strings("file name", ".dat" ("string")) -> (w40:string)
      n14 = String To Path(string=w40) -> (path=w32:path)
      n15 = Concatenate Strings("Time (s)", w26, "DC Voltage (V)" ("string"), w26, "dI (A)" ("string"), w26, "dV (V)" ("string"), w26, "Differential Conductance dI/dV (S)", w26, "Source Voltage (V)", w26, "DC Current (A)", "\r\n") -> (w41:string)
      n16 = Build Path(base path="Folder", name or relative path=w32) -> (appended path=w31:path)
      n17 = flat-sequence {
        tunnel: w31 -> [w47]
        tunnel: w41 -> [w50]
        tunnel: [w50] -> w43
        tunnel: [w49] -> w38
        tunnel: [w48] -> w42
        tunnel: w43 -> [w57]
        tunnel: w42 -> [w56]
        frame #0 {
          n18 = Open/Create/Replace File(file path (use dialog)=w47, operation (0:open)=T2."create") -> (error out=w46:errorcluster)  [unwired: 4 in, 2 out]
          n19 = Unbundle By Name(w46) -> ("status"=w44:bool)
          n20 = case shown="True" w44 {
            tunnel: [FALSE ("Yes") w54] -> w49
            tunnel: [w51 w53] -> w48
            tunnel: w47 -> [w51 w53]
            frame False {
            }
            frame True {
              n21 = call "Message to User"() -> ("Yes"=w55:bool)  [unwired: 10 in, 1 out]
              n22 = Not(x=w55) -> (.not. x?=w54:bool)
            }
          }
        }
        frame #1 {
          n23 = call <vilib>:"Write Characters To File.vi"("append to file? (new file:F)"=TRUE, "character string"=w57, "file path (dialog if empty)"=w56) -> ()  [unwired: 2 in, 1 out]
          "File path" <- w56
        }
      }
      n24 = Stop(stop? (T)=w38) -> ()
    }
    frame #4 {
      n25 = Wait (ms)(milliseconds to wait=u32 1000) -> ()  [unwired: 1 out]
    }
    frame #5 {
      n26 = flat-sequence {
        tunnel: [w73] -> w61
        tunnel: [w72] -> _
        tunnel: cluster{dbl, "Field Reading":dbl}[] [] -> [w75]
        tunnel: w63 -> [w74]
        frame #0 {
          n27 = local read "MFLI Address"() -> (w69:string)
          n28 = local read "Keithley 2636B (channelA)"() -> (w65:refnum<visa-resource-name>)
          n29 = call "ziOpen.vi"("Address"=w69) -> ("Error Out"=w68:errorcluster, "HandleOut"=w71:T3)  [unwired: 3 in, 1 out]
          n30 = call "ziCheckVersion.vi"("Handle In"=w71, "Error In"=w68) -> ("Handle Out"=w70:T3, "Error Out"=w67:errorcluster)  [unwired: 11 in, 1 out]
          n31 = for {
            tunnel: "From" -> [w88] mode=indexing
            tunnel: "To" -> [w87] mode=indexing
            tunnel: "Step" -> [w86] mode=indexing
            shift-right: [w90] -> w72
            shift-left: w75 -> [w91]
            tunnel: w74 -> [w85]
            shift-right: [w83] -> w66
            shift-left: w70 -> [w84]
            shift-right: [w82] -> w73
            shift-left: w67 -> [w81]
            shift-right: [w79] -> _
            shift-left: w65 -> [w80]
            n32 = call "Build_serie_EL.vi"("end value"=w87, "increment"=w86, "start value"=w88) -> ("output array"=w89:dbl[])
            n33 = for {
              tunnel: w89 -> [w101] mode=indexing
              shift-right: [w99] -> w90
              shift-left: w91 -> [w100]
              tunnel: w85 -> [w98]
              shift-right: [w96] -> w83
              shift-left: w84 -> [w97]
              shift-right: [w95] -> w82
              shift-left: w81 -> [w94]
              shift-right: [w92] -> w79
              shift-left: w80 -> [w93]
              n34 = stacked-sequence {
                tunnel: w100 -> [_ _ w162]
                tunnel: w101 -> [w106 _ _]
                tunnel: [_ _ w161] -> w99
                tunnel: w98 -> [_ _ w158]
                tunnel: w97 -> [w102 _ w154]
                tunnel: [_ _ w153] -> w96
                tunnel: [_ _ w152] -> w95
                tunnel: w94 -> [w103 _ w151]
                tunnel: w93 -> [w104 _ _]
                tunnel: [w105 _ _] -> w92
                frame #0 {
                  n35 = flat-sequence {
                    tunnel: w106 -> [w113]
                    tunnel: [w112] -> w105
                    tunnel: w104 -> [w111]
                    tunnel: w103 -> [w117]
                    tunnel: w102 -> [w116]
                    frame #0 {
                      w110 = 0
                      w109 = 1
                      n36 = call-poly "Configure Source.vi"("VISA resource name"=w111, "Source Measure Unit Channel (0: Channel A)"=w110, "Range Type (1: Voltage)"=w109, "Auto Range (T: Enable)"=TRUE) -> ("VISA resource name out"=w107:refnum<visa-resource-name>)  [unwired: 10 in, 1 out]
                      n37 = call "Configure Source (Level).vi"("VISA resource name"=w107, "Source Measure Unit Channel (0: Channel A)"=w110, "Level Type (1: Voltage)"=w109, "Voltage Level (0 V)"=w113) -> ("VISA resource name out"=w112:refnum<visa-resource-name>)  [unwired: 10 in, 1 out]
                      "Vset (V)" <- w113
                    }
                    frame #1 {
                      n38 = Wait (ms)(milliseconds to wait=50) -> ()  [unwired: 1 out]
                    }
                    frame #2 {
                      n39 = case shown="True" "MFLI Autorange" {
                        tunnel: w117 -> [_ w119]
                        tunnel: w116 -> [_ w118]
                        frame False {
                        }
                        frame True {
                          n40 = call-poly "ziSetValue.vi"("Error In"=w119, "Value"=1.0, "Path"="sigins/0/autorange", "Handle In"=w118) -> ("Error Out"=w125:errorcluster, "Handle Out"=w124:T3)  [unwired: 1 in]
                          n41 = call-poly "ziSetValue.vi"("Error In"=w125, "Value"=1.0, "Path"="currins/0/autorange", "Handle In"=w124) -> ("Error Out"=w127:errorcluster, "Handle Out"=w126:T3)  [unwired: 1 in]
                          n42 = call "ziSync.vi"("Handle In"=w126, "Error In"=w127) -> ()  [unwired: 12 in, 2 out]
                        }
                      }
                    }
                  }
                }
                frame #1 {
                  n43 = Multiply(x="Delay (s)", y=1000) -> (x*y=w129:dbl)
                  n44 = Wait (ms)(milliseconds to wait=w129) -> ()  [unwired: 1 out]
                }
                frame #2 {
                  n45 = Tick Count (ms)() -> (millisecond timer value=w159:u32)
                  n46 = Subtract(x=w159, y=w158) -> (x-y=w157:u32)
                  n47 = flat-sequence {
                    tunnel: [w169] -> w145
                    tunnel: [w168] -> w144
                    tunnel: w151 -> [w170]
                    tunnel: w154 -> [w171]
                    tunnel: [w165] -> w133
                    tunnel: "MFLI Average" -> [w164]
                    tunnel: [w164] -> w131
                    tunnel: w145 -> [w187]
                    tunnel: w144 -> [w186]
                    tunnel: [w185] -> w143
                    tunnel: [w184] -> w142
                    tunnel: [w180] -> w141
                    tunnel: [w183] -> w140
                    tunnel: w133 -> [w183]
                    tunnel: w131 -> [w179]
                    tunnel: [w200] -> w136
                    tunnel: [w201] -> w137
                    tunnel: [w202] -> w152
                    tunnel: [w203] -> w153
                    tunnel: w143 -> [w203]
                    tunnel: w142 -> [w202]
                    tunnel: w141 -> [w201]
                    tunnel: w140 -> [w200]
                    tunnel: [w197] -> w135
                    tunnel: [w195] -> _
                    frame #0 {
                      n48 = for {
                        N: w164 -> [_]
                        tunnel: [w172] -> w167 mode=indexing
                        shift-right: [w174] -> w169
                        shift-left: w171 -> [w176]
                        shift-right: [w173] -> w168
                        shift-left: w170 -> [w175]
                        n49 = call-poly "ziGetValue.vi"("error in"=w175, "Path"="demods/0/sample", "Handle In"=w176) -> ("error out"=w173:errorcluster, "Demod Sample Out"=w177:T1, "Handle Out"=w174:T3)
                        "Demod Sample Out" <- w177
                        n50 = Unbundle By Name(w177) -> ("X (Vrms)"=w172:dbl)  [unwired: 2 out]
                      }
                      n51 = Add Array Elements(numeric array=w167) -> (sum=w166:dbl)
                      n52 = Divide(x=w166, y=w164) -> (x/y=w165:dbl)
                    }
                    frame #1 {
                      n53 = for {
                        N: w179 -> [_]
                        tunnel: [w188] -> w181 mode=indexing
                        shift-right: [w190] -> w185
                        shift-left: w187 -> [w192]
                        shift-right: [w189] -> w184
                        shift-left: w186 -> [w191]
                        n54 = call-poly "ziGetValue.vi"("error in"=w191, "Path"="demods/2/sample", "Handle In"=w192) -> ("error out"=w189:errorcluster, "Demod Sample Out"=w193:T1, "Handle Out"=w190:T3)
                        "Demod Sample Out 2" <- w193
                        n55 = Unbundle By Name(w193) -> ("X (Vrms)"=w188:dbl)  [unwired: 2 out]
                      }
                      n56 = Add Array Elements(numeric array=w181) -> (sum=w182:dbl)
                      n57 = Divide(x=w182, y=w179) -> (x/y=w180:dbl)
                    }
                    frame #2 {
                      n58 = local read "Nanovoltmeter 2182a VISA"() -> (w195:refnum<visa-resource-name>)
                      n59 = for {
                        N: "DC Voltage averaging" -> [_]
                        tunnel: [w205] -> w198 mode=indexing
                        shift-right: [w204] -> _
                        shift-left: w195 -> [w206]
                        n60 = call "Get-V_K2182A_VISA_EL.vi"("VISA K2182A"=w206) -> ("V (V)"=w205:dbl, "VISA K2182A"=w204:refnum<visa-resource-name>)  [unwired: 2 in, 1 out]
                      }
                      n61 = Add Array Elements(numeric array=w198) -> (sum=w199:dbl)
                      n62 = Divide(x=w199, y="DC Voltage averaging") -> (x/y=w197:dbl)
                      "DC Voltage (V)" <- w197
                    }
                  }
                  n63 = Divide(x=w157, y=1000) -> (x/y=w155:dbl)
                  "Time(s)" <- w155
                  n64 = local read "Vset (V)"() -> (w138:dbl)
                  n65 = Divide(x=w137, y=w136) -> (x/y=w160:dbl)
                  "dI/dV (S)" <- w160
                  n66 = Divide(x=w138, y="Resistance used for DC (ohm)") -> (x/y=w134:dbl)
                  n67 = Bundle(w135, w160) -> (w163:cluster{dbl, dbl})  [unwired: 1 in]
                  n68 = Build Array(w155, w135, w137, w136, w160, w138, w134) -> (w146:dbl[])
                  "data" <- w146
                  n69 = Build Array (concatenate)(w162, w163) -> (w161:cluster{dbl, "Field Reading":dbl}[])
                  "dI/dV vs DC Bias (V)" <- w161
                  n70 = local read "File path"() -> (w148:path)
                  n71 = Array To Spreadsheet String(array=w146, 3:"%e" ("format string")) -> (spreadsheet string=w149:string)  [unwired: 1 in]
                  n72 = call <vilib>:"Write Characters To File.vi"("append to file? (new file:F)"=TRUE, "character string"=w149, "file path (dialog if empty)"=w148) -> ()  [unwired: 2 in, 1 out]
                  "dI (A)" <- w137
                  "dV (V)" <- w136
                }
              }
            }
          }
          n73 = call "ziClose.vi"("Handle In"=w66) -> ()  [unwired: 1 in, 4 out]
        }
      }
      n74 = Unbundle By Name(w61) -> ("status"=w60:bool)
      n75 = Or(x=w60, y="stop") -> ()  [unwired: 1 out]
    }
    frame #6 {
      w208 = 0
      n76 = call "Configure Source (Level).vi"("VISA resource name"=w209, "Source Measure Unit Channel (0: Channel A)"=w208, "Level Type (1: Voltage)"=1, "Voltage Level (0 V)"=0.0) -> ("VISA resource name out"=w212:refnum<visa-resource-name>)  [unwired: 10 in, 1 out]
      n77 = call "Enable Source Output.vi"("Output Mode (0: Turn off)"=w208, "Source Measure Unit Channel (0: Channel A)"=w208, "VISA resource name"=w212) -> ("VISA resource name out"=w207:refnum<visa-resource-name>)  [unwired: 7 in, 1 out]
      n78 = call "Close.vi"("VISA resource name"=w207) -> ()  [unwired: 10 in, 1 out]
    }
  }
